vi "SetColors.vi"(8 "error in (no error)":errorcluster, 10 "Colors":T1={"Top Color"=16448250, "Left Color"=16448250, "Center Color"=16448250, "Right Color"=16448250, "Bottom Color"=16448250}, 11 "PentaPanesGUI in":refnum<class "PentaPanes.lvclass">) -> (0 "error out":errorcluster, 3 "PentaPanesGUI out":refnum<class "PentaPanes.lvclass">)   [LabVIEW 2022 SP3, in "PentaPanesLibrary.lvlib" / "PentaPanes.lvclass"]
doc: "SetColors\nThis VI Sets the BG color of all the panes. \n\nColors - a structure that contains RGB colors for each pane"
uses:
  PentaPanes.lvclass
  PanesColors.ctl
  PentaPanes.lvclass/PentaPanes.ctl
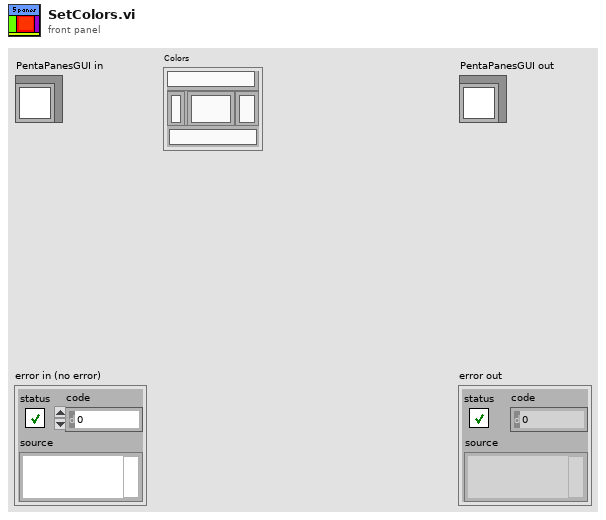
[diagram p1: front panel]
types:
  T1 = typedef "PentaPanesLibrary.lvlib/PentaPanes.lvclass/PanesColors.ctl" = cluster{"Top Color":u32, "Left Color":u32, "Center Color":u32, "Right Color":u32, "Bottom Color":u32}
  T2 = typedef "PentaPanesLibrary.lvlib/PentaPanes.lvclass/PanesCluster.ctl" = cluster{"Top Pane":refnum<vi>, "Left Pane":refnum<vi>, "Center Pane":refnum<vi>, "Right Pane":refnum<vi>, "Bottom Pane":refnum<vi>}
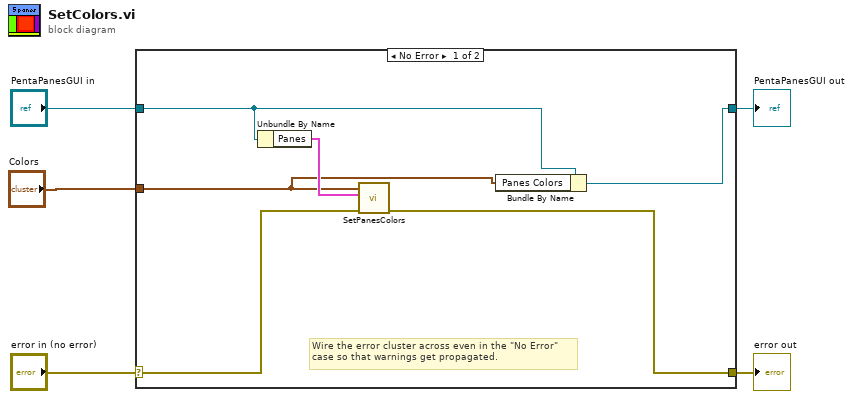
[diagram p0: block diagram]
diagram:
  n1 = case shown="No Error" "error in (no error)" {
    selector: "error in (no error)" -> [w10 w13]
    tunnel: [w9 w13] -> w4
    tunnel: [w7 w12] -> w2
    tunnel: "PentaPanesGUI in" -> [w8 w12]
    tunnel: "Colors" -> [w6 _]
    frame No Error {
      # "Wire the error cluster across even in the \"No Error\"\ncase so that warnings get propagated."
      n2 = Unbundle By Name(w8) -> ("Panes"=w11:T2)
      n3 = call "SetPanesColors.vi"("error in (no error)"=w10, "Panes"=w11, "Colors"=w6) -> ("error out"=w9:errorcluster)  [unwired: 8 in]
      n4 = Bundle By Name(cluster=w8, "Panes Colors"=w6) -> (w7:refnum<class "PentaPanes.lvclass">)
    }
    frame Error {
    }
  }
  "error out" <- w4
  "PentaPanesGUI out" <- w2
